vi "rspvtd_Timeout.vi"(8 "error in":errorcluster, 11 "Data in":variant) -> (0 "error out":errorcluster, 3 "Data out":T1={"Data"=variant(string ""), "Auxiliary"=variant})   [LabVIEW 2018, in "Work Planer.lvclass"]
doc: "This VI converts variant data contained in the associated <b>Public API Response</b> message to its correct data type.\n---"
uses:
  Work Planer.lvclass
  rsp_Timeout.ctl
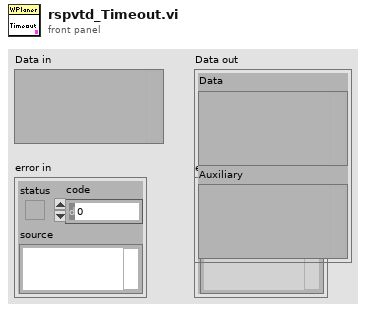
[diagram p1: front panel]
types:
  T1 = typedef "Work Planer.lvclass/rsp_Timeout.ctl" = cluster{"Data":variant, "Auxiliary":variant}
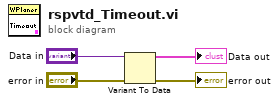
[diagram p0: block diagram]
diagram:
  n1 = Variant To Data(error in="error in", Variant="Data in") -> (data=→"Data out":T1, error out=→"error out":errorcluster)  [unwired: 1 in]
